vi "Start Log.vi"(8 "error in (no error)":errorcluster, 9 "Timestamp":string, 10 "Series":string, 11 "LoggingHandler in":refnum<class "LoggingHandler.lvclass">) -> (0 "error out":errorcluster, 3 "LoggingHandler out":refnum<class "LoggingHandler.lvclass">)   [LabVIEW 2020, in "VolatusDataLogger.lvlib" / "LoggingHandler.lvclass"]
uses:
  LoggingHandler.lvclass
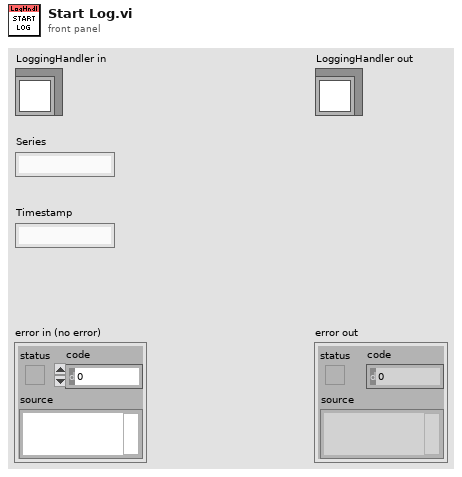
[diagram p1: front panel]
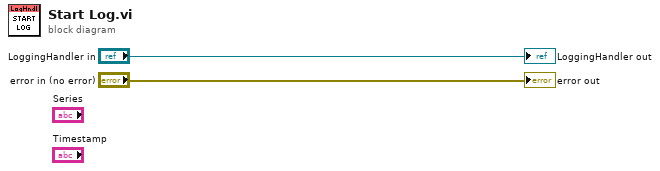
[diagram p0: block diagram]
diagram:
  "error out" <- "error in (no error)"
  "LoggingHandler out" <- "LoggingHandler in"
